vi "json_parse_array.vi"(8 "error in (no error)":errorcluster, 10 "parent key":string, 11 "data":string) -> (0 "error out":errorcluster, 2 "pairs":cluster{"key":string, "value":variant}[](array[cluster]), 3 "remaining data":string)   [LabVIEW 2017]
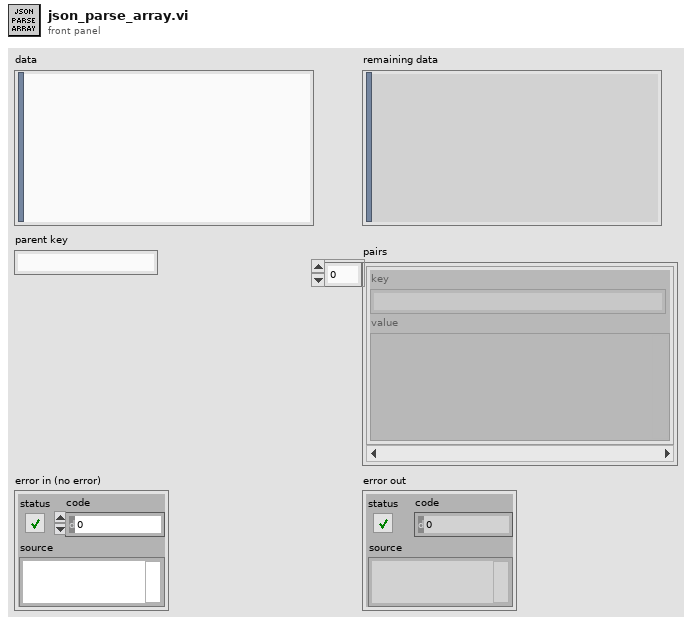
[diagram p1: front panel]
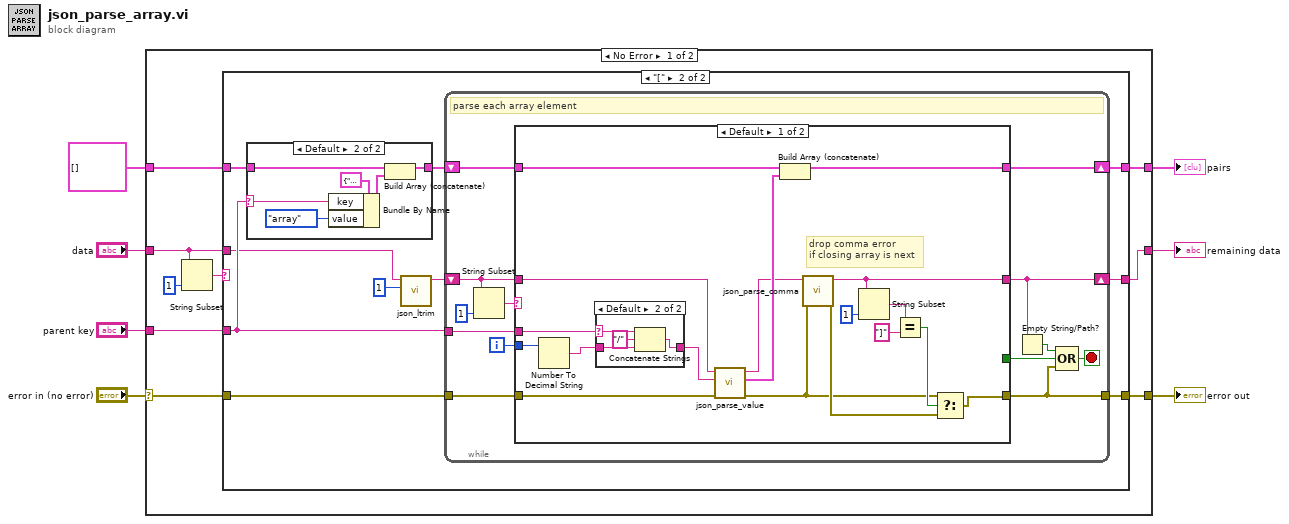
[diagram p0: block diagram]
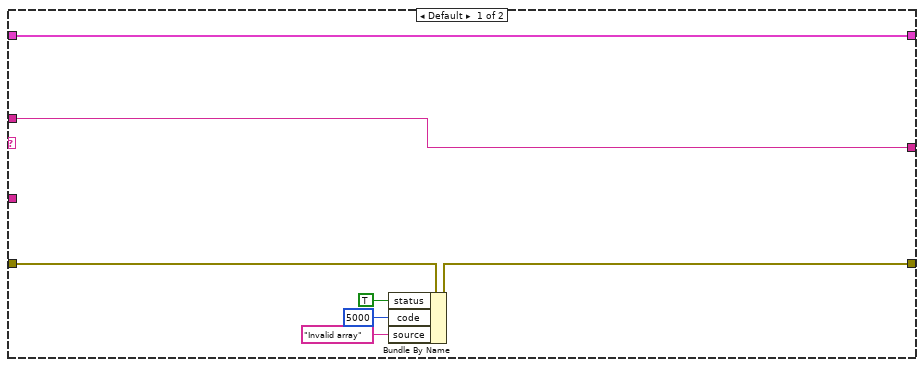
[diagram p2: hidden frame]
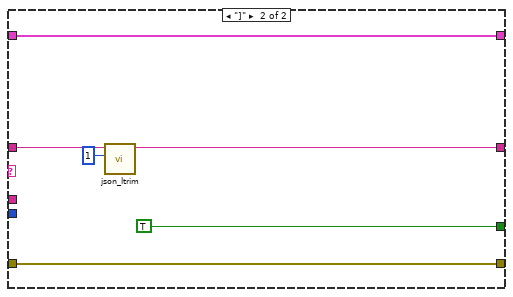
[diagram p5: hidden frame]
diagram:
  n1 = case shown="No Error" "error in (no error)" {
    selector: "error in (no error)" -> [w15 w85]
    tunnel: [w16 w84] -> w7
    tunnel: [w14 w85] -> w5
    tunnel: "parent key" -> [w13 _]
    tunnel: [w12 w83] -> w3
    tunnel: cluster{"key":string, "value":variant}[] [] ("appended array") -> [w11 w84]
    tunnel: "data" -> [w10 w83]
    frame No Error {
      n2 = String Subset(string=w10, length (rest)=1 ("length (rest)")) -> (substring=w9:string)  [unwired: 1 in]
      n3 = case shown="\"[\"" w9 {
        tunnel: w10 -> [w23 w26]
        tunnel: [w23 w30] -> w12
        tunnel: [w22 w33] -> w16
        tunnel: w11 -> [w22 w27]
        tunnel: w15 -> [w21 w32]
        tunnel: [w20 w31] -> w14
        tunnel: w13 -> [_ w28]
        frame Default {
          n4 = Bundle By Name(cluster=w21, "status"=TRUE, "code"=5000, "source"="Invalid array") -> (w20:errorcluster)
        }
        frame "[" {
          n5 = case shown="Default" w28 {
            selector: w28 -> [_ w37]
            tunnel: [w34 w38] -> w29
            tunnel: w27 -> [w34 w36]
            frame "" {
            }
            frame Default {
              n6 = Bundle By Name(cluster=cluster{"key":string, "value":variant} {"key"="", "value"=variant} ("pair"), "key"=w37, "value"=enum8{"array"}."array" ("array")) -> (w39:cluster{"key":string, "value":variant})
              n7 = Build Array (concatenate)(w36, w39) -> (w38:cluster{"key":string, "value":variant}[])
            }
          }
          n8 = call "json_ltrim.vi"("offset (0)"=1 ("length (rest)"), "data"=w26) -> ("left trim whitespace"=w25:string)  [unwired: 9 in]
          n9 = while {
            shift-right: [w53] -> w33
            shift-left: w29 -> [w52]
            shift-right: [w46] -> w30
            shift-left: w25 -> [w44]
            tunnel: w32 -> [w51]
            tunnel: [w47] -> w31
            tunnel: w28 -> [w50]
            i -> [w41]
            stop <- w48 stop-if-true
            # "parse each array element"
            n10 = String Subset(string=w44, length (rest)=1 ("length (rest)")) -> (substring=w43:string)  [unwired: 1 in]
            n11 = case shown="Default" w43 {
              tunnel: [_ TRUE] -> w49
              tunnel: [w71 w81] -> w53
              tunnel: w52 -> [w70 w81]
              tunnel: w44 -> [w67 w78]
              tunnel: [w55 w77] -> w46
              tunnel: w51 -> [w68 w80]
              tunnel: [w57 w80] -> w47
              tunnel: w50 -> [w69 _]
              tunnel: w41 -> [w64 _]
              frame Default {
                # "drop comma error\nif closing array is next"
                n12 = Number To Decimal String(number=w64) -> (decimal integer string=w63:string)  [unwired: 1 in]
                n13 = case shown="Default" w69 {
                  selector: w69 -> [_ w76]
                  tunnel: w63 -> [w72 w75]
                  tunnel: [w72 w74] -> w66
                  frame "" {
                  }
                  frame Default {
                    n14 = Concatenate Strings(w76, "/" ("format string"), w75) -> (w74:string)
                  }
                }
                n15 = call "json_parse_value.vi"("error in (no error)"=w68, "key"=w66, "data"=w67) -> ("error out"=w54:errorcluster, "pairs"=w65:cluster{"key":string, "value":variant}[], "remaining data"=w56:string)  [unwired: 6 in]
                n16 = Build Array (concatenate)(w70, w65) -> (w71:cluster{"key":string, "value":variant}[])
                n17 = call "json_parse_comma.vi"("error in (no error)"=w54, "data"=w56) -> ("error out"=w58:errorcluster, "remaining data"=w55:string)  [unwired: 8 in]
                n18 = String Subset(string=w55, length (rest)=1 ("length (rest)")) -> (substring=w61:string)  [unwired: 1 in]
                n19 = Equal?(x=w61, y="]") -> (x = y?=w59:bool)
                n20 = Select(t=w54, s=w59, f=w58) -> (s? t:f=w57:errorcluster)
              }
              frame "]" {
                n21 = call "json_ltrim.vi"("offset (0)"=1 ("length (rest)"), "data"=w78) -> ("left trim whitespace"=w77:string)  [unwired: 9 in]
              }
            }
            n22 = Empty String/Path?(string/path=w46) -> (empty?=w45:bool)
            n23 = Compound Arithmetic op=OR(w45, w49, w47) -> (w48:bool)
          }
        }
      }
    }
    frame Error {
    }
  }
  "remaining data" <- w3
  "pairs" <- w7
  "error out" <- w5
